vi "closeImaqSession.vi"(8 "error in":errorcluster, 10 "Updated camera":T2, 11 "Saving":bool) -> (0 "error out":errorcluster, 2 "Updated camera out":T2)   [LabVIEW 2017]
uses:
  <vilib>/vision/Image Controls.llb/IMAQ Image.ctl
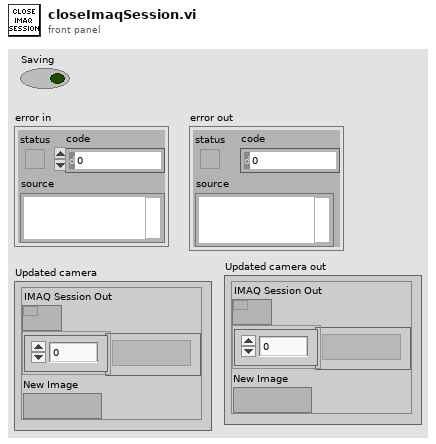
[diagram p1: front panel]
types:
  T1 = typedef "IMAQ Image.ctl" = refnum<image>
  T2 = cluster{"IMAQ Session Out":refnum<k11>, "Array":T1[], "New Image":T1}
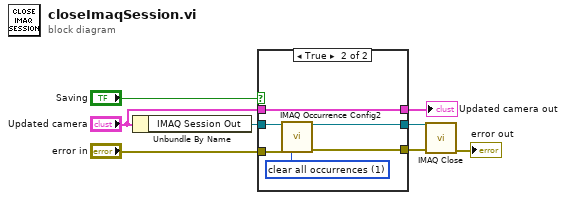
[diagram p0: block diagram]
diagram:
  n1 = Unbundle By Name("Updated camera") -> ("IMAQ Session Out"=w7:refnum<k11>)
  n2 = case shown="True" "Saving" {
    tunnel: w7 -> [w11 w17]
    tunnel: "error in" -> [w10 w15]
    tunnel: [w11 w14] -> w5
    tunnel: [w10 w13] -> w4
    tunnel: "Updated camera" -> [w9 w12]
    tunnel: [w9 w12] -> w1
    frame False {
    }
    frame True {
      w16 = u16 1 items=["create an occurrence", "clear all occurrences"] ("create/clear")
      n3 = call <vilib>:"IMAQ Occurrence Config2.vi"("IMAQ Session In"=w17, "error in (no error)"=w15, "create/clear"=w16) -> ("IMAQ Session Out"=w14:refnum<k11>, "error out"=w13:errorcluster)  [unwired: 10 in, 1 out]
    }
  }
  "Updated camera out" <- w1
  n4 = call <vilib>:"IMAQ Close.vi"("error in (no error)"=w4, "IMAQ Session In"=w5) -> ("error out"=→"error out":errorcluster)  [unwired: 9 in]
